vi "getColorIndex.vi"(11 "Color":u32(colorbox)) -> (3 "excel color table index":i16)   [LabVIEW 2017, in "LabVIEW NPOI.lvlib" / "MS-Excel.lvclass"]
uses:
  MS-Excel.lvclass
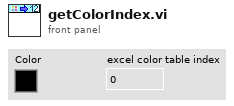
[diagram p1: front panel]
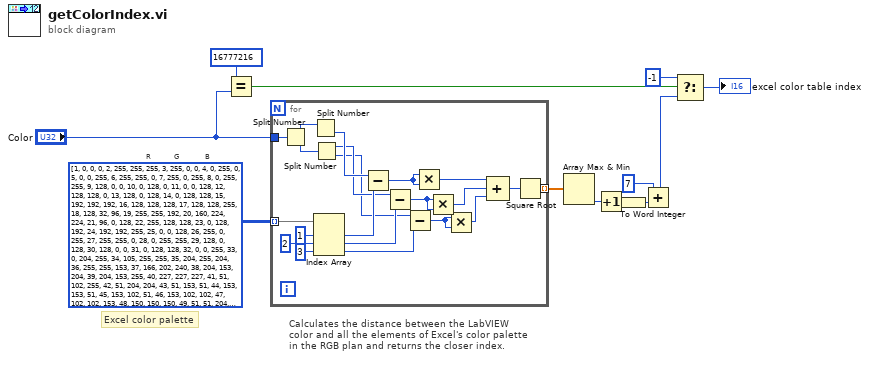
[diagram p0: block diagram]
diagram:
  # "Calculates the distance between the LabVIEW color and all the elements of Excel's color palette in the RGB plan and returns the closer index."
  # "B"
  # "G"
  # "R"
  # "Excel color palette"
  n1 = Equal?(x=16777216, y="Color") -> (x = y?=w8:bool)
  n2 = for {
    tunnel: i32[][] [[1, 0, 0, 0], [2, 255, 255, 255], [3, 255, 0, 0], [4, 0, 255, 0], [5, 0, 0, 255], [6, 255, 255, 0], [7, 255, 0, 255], [8, 0, 255, 255], [9, 128, 0, 0], [10, 0, 128, 0], [11, 0, 0, 128], [12, 128, 128, 0], [13, 128, 0, 128], [14, 0, 128, 128], [15, 192, 192, 192], [16, 128, 128, 128], [17, 128, 128, 255], [18, 128, 32, 96], [19, 255, 255, 192], [20, 160, 224, 224], [21, 96, 0, 128], [22, 255, 128, 128], [23, 0, 128, 192], [24, 192, 192, 255], [25, 0, 0, 128], [26, 255, 0, 255], [27, 255, 255, 0], [28, 0, 255, 255], [29, 128, 0, 128], [30, 128, 0, 0], [31, 0, 128, 128], [32, 0, 0, 255], [33, 0, 204, 255], [34, 105, 255, 255], [35, 204, 255, 204], [36, 255, 255, 153], [37, 166, 202, 240], [38, 204, 153, 204], [39, 204, 153, 255], [40, 227, 227, 227], [41, 51, 102, 255], [42, 51, 204, 204], [43, 51, 153, 51], [44, 153, 153, 51], [45, 153, 102, 51], [46, 153, 102, 102], [47, 102, 102, 153], [48, 150, 150, 150], [49, 51, 51, 204], [50, 51, 102, 102], [51, 0, 51, 0], [52, 51, 51, 0], [53, 102, 51, 0], [54, 153, 51, 102], [55, 51, 51, 153], [56, 66, 66, 66]] ("data") -> [w31] mode=indexing
    tunnel: [w13] -> w12 mode=indexing
    tunnel: "Color" -> [w20]
    n3 = Split Number(x=w20) -> (hi(x)=w33:u16, lo(x)=w32:u16)
    n4 = Split Number(x=w33) -> (lo(x)=w24:u8)  [unwired: 1 out]
    n5 = Split Number(x=w32) -> (hi(x)=w23:u8, lo(x)=w22:u8)
    n6 = Index Array(array=w31, index #1=1 ("Index"), index #2=2 ("Index"), index #3=3 ("Index")) -> (element #1=w25:i32, element #2=w26:i32, element #3=w27:i32)
    n7 = Subtract(x=w24, y=w25) -> (x-y=w19:i32)
    n8 = Subtract(x=w23, y=w26) -> (x-y=w17:i32)
    n9 = Subtract(x=w22, y=w27) -> (x-y=w18:i32)
    n10 = Multiply(x=w19, y=w19) -> (x*y=w16:i32)
    n11 = Multiply(x=w17, y=w17) -> (x*y=w15:i32)
    n12 = Multiply(x=w18, y=w18) -> (x*y=w14:i32)
    n13 = Compound Arithmetic op=ADD(w16, w15, w14) -> (w21:i32)
    n14 = Square Root(x=w21) -> (sqrt(x)=w13:dbl)
  }
  n15 = Array Max & Min(array=w12) -> (min index (indices)=w11:i32)  [unwired: 3 out]
  n16 = Increment(x=w11) -> (x+1=w7:i32)
  n17 = To Word Integer(number=w7) -> (16bit integer=w3:i16)
  n18 = Add(x=i16 7, y=w3) -> (x+y=w2:i16)
  n19 = Select(t=i16 -1, s=w8, f=w2) -> (s? t:f=→"excel color table index":i16)
